vi "serialize_mmWaveMoves.vi"(10 "Moves":T1[](array[typedef])) -> (2 "Moves string":string)   [LabVIEW 2018]
uses:
  APARMainSubvis/VXM Public API/singleAxisMoveDef.ctl
  APARMainSubvis/VXM Public API/mmWaveAxis.ctl
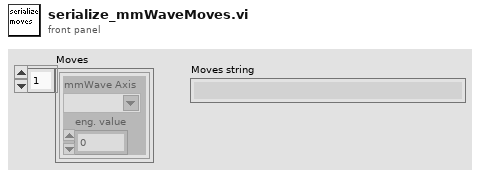
[diagram p1: front panel]
types:
  T1 = typedef "singleAxisMoveDef.ctl" = cluster{"mmWave Axis":T2, "eng. value":dbl}
  T2 = typedef "mmWaveAxis.ctl" = string
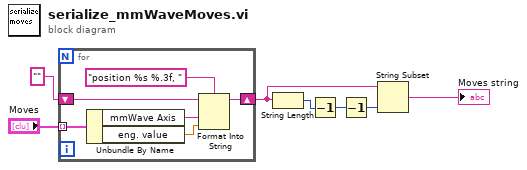
[diagram p0: block diagram]
diagram:
  n1 = for {
    tunnel: "Moves" -> [w13] mode=indexing
    shift-right: [w8] -> w3
    shift-left: "" -> [w9]
    n2 = Unbundle By Name(w13) -> ("mmWave Axis"=w11:T2, "eng. value"=w10:dbl)
    n3 = Format Into String(format string="position %s %.3f, ", initial string=w9, w11, w10) -> (resulting string=w8:string)  [unwired: 1 in, 1 out]
  }
  n4 = String Length(string=w3) -> (length=w5:i32)
  n5 = Decrement(x=w5) -> (x-1=w4:i32)
  n6 = Decrement(x=w4) -> (x-1=w1:i32)
  n7 = String Subset(string=w3, length (rest)=w1) -> (substring=→"Moves string":string)  [unwired: 1 in]
